vi "TextToSpeech.vi"(9 "Text To Be Spoken":string="LabVIEW is the greatest software ever to be created. ", 10 "Choose a Voice":i32(ring)=1 items=["Microsoft David Desktop - English (United States)", "Microsoft Zira Desktop - English (United States)"], 11 "SpeechLib.ISpeechVoice":refnum<k7>) -> (0 "error out":errorcluster, 3 "SpeechLib.ISpeechVoice 2":refnum<k7>)   [LabVIEW 2018]
doc: "This VI is an example of Text to Speech (TTS) using the Microsoft Speech SDK 5.1. Turn off all audio applications before running this VI.\n\n1. Enter the text to be read in the text box.\n2. Choose a voice.\n3. Run the VI.\n\nNote: The first time you run this VI, the ring control might change according to the voice order that the Speech SDK installed it in. This varies on different systems. But after the first time, the ring control remains the same.\n\nFor more information on the methods and properties, refer to the documentation that is included with the SDK or visit www.microsoft.com/speech."
panel:
  # "Overview: This example uses Microsoft Speech SDK to convert text into audible speech .\nRequirements: LabVIEW 2012 (or compatible)\nInstructions: \n1. Set Choose a Voice and Text To Be Spoken controls\n2. Run the VI"
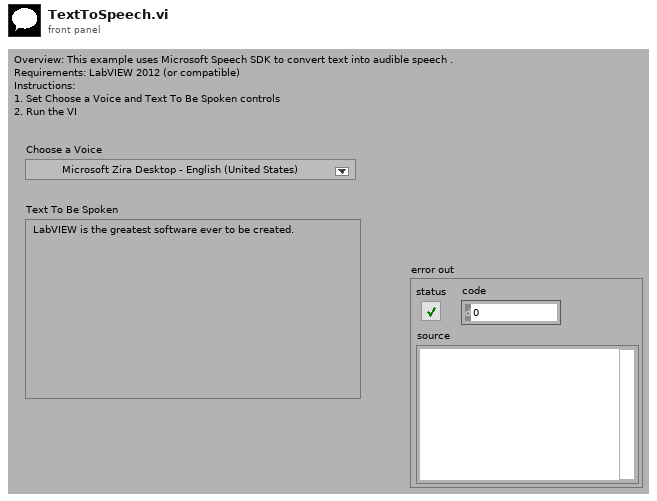
[diagram p1: front panel]
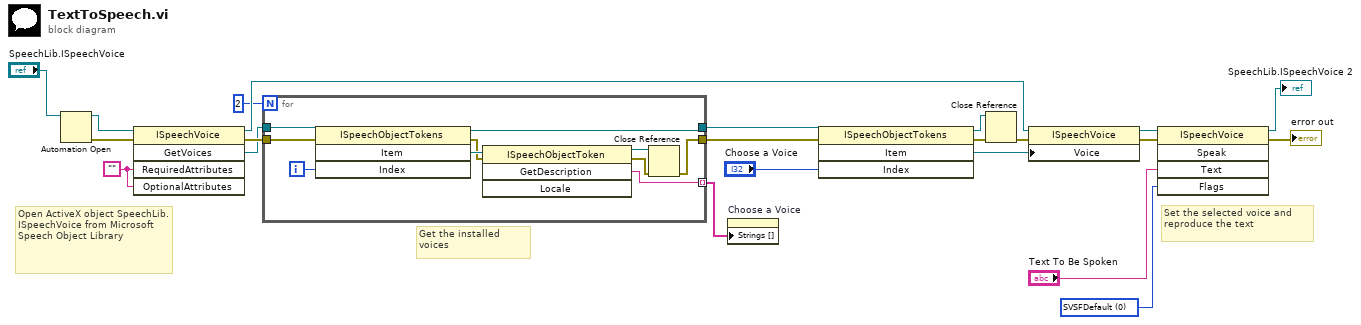
[diagram p0: block diagram]
diagram:
  w13 = ""
  w20 = 0 items=["SVSFDefault"=0, "SVSFlagsAsync"=1, "SVSFPurgeBeforeSpeak"=2, "SVSFIsFilename"=4, "SVSFIsXML"=8, "SVSFIsNotXML"=16, "SVSFPersistXML"=32, "SVSFNLPSpeakPunc, SVSFNLPMask"=64, "SVSFVoiceMask"=127, "SVSFUnusedFlags"=-128] ("Flags")
  # "Set the selected voice and reproduce the text"
  # "Get the installed voices"
  # "Open ActiveX object SpeechLib.ISpeechVoice from Microsoft Speech Object Library"
  n1 = Automation Open(Automation Refnum="SpeechLib.ISpeechVoice") -> (Automation Refnum=w21:refnum<k7>, error out=w12:errorcluster)  [unwired: 1 in, 2 out]
  n2 = invoke class="ISpeechVoice" method="GetVoices"(reference=w21, error in=w12, "RequiredAttributes"=w13, "OptionalAttributes"=w13) -> (reference out=w18:refnum<k7>, error out=w11:errorcluster, "GetVoices"=w10:refnum<k7>)  [unwired: 1 in, 2 out]
  n3 = for {
    N: 2 -> [_]
    tunnel: [w23] -> w4
    tunnel: w11 -> [w29]
    tunnel: w10 -> [w28]
    tunnel: [w27] -> w8
    tunnel: [w26] -> w7 mode=indexing
    i -> [w31]
    n4 = invoke class="ISpeechObjectTokens" method="Item"(reference=w28, error in=w29, "Index"=w31) -> (reference out=w27:refnum<k7>, error out=w25:errorcluster, "Item"=w32:refnum<k7>)  [unwired: 1 in, 1 out]
    n5 = invoke class="ISpeechObjectToken" method="GetDescription"(reference=w32, error in=w25) -> (reference out=w30:refnum<k7>, error out=w24:errorcluster, "GetDescription"=w26:string)  [unwired: 2 in, 1 out]
    n6 = Close Reference(reference=w30, error in (no error)=w24) -> (error out=w23:errorcluster)
  }
  n7 = property on="Choose a Voice" class="Ring (strict)"("Strings []"=w7) -> ()  [unwired: 2 in, 2 out]
  n8 = invoke class="ISpeechObjectTokens" method="Item"(reference=w8, error in=w4, "Index"="Choose a Voice") -> (reference out=w5:refnum<k7>, error out=w3:errorcluster, "Item"=w14:refnum<k7>)  [unwired: 1 in, 1 out]
  n9 = Close Reference(reference=w5, error in (no error)=w3) -> (error out=w2:errorcluster)
  n10 = property class="ISpeechVoice"(reference=w18, error in=w2, "Voice"=w14) -> (reference out=w17:refnum<k7>, error out=w16:errorcluster)
  n11 = invoke class="ISpeechVoice" method="Speak"(reference=w17, error in=w16, "Text"="Text To Be Spoken", "Flags"=w20) -> (reference out=→"SpeechLib.ISpeechVoice 2":refnum<k7>, error out=→"error out":errorcluster)  [unwired: 1 in, 3 out]
